vi "Write Optimum Mixer Level for IMD.vi"(10 "Optimum Mixer Level for IMD":T1(array[cluster]), 11 "Spectrum Analyzer in":refnum<class "Spectrum Analyzer.lvclass">) -> (3 "Spectrum Analyzer out":refnum<class "Spectrum Analyzer.lvclass">)   [LabVIEW 2020, in "Spectrum Analyzer.lvclass"]
uses:
  Spectrum Analyzer.lvclass
  Spectrum Analyzer.lvclass/Spectrum Analyzer.ctl
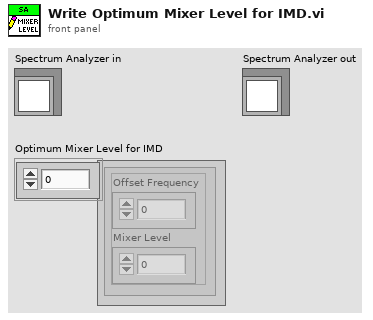
[diagram p1: front panel]
types:
  T1 = cluster{"Offset Frequency":dbl, "Mixer Level":dbl}[]
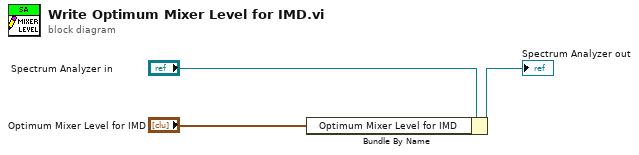
[diagram p0: block diagram]
diagram:
  n1 = Bundle By Name(cluster="Spectrum Analyzer in", "Optimum Mixer Level for IMD"="Optimum Mixer Level for IMD") -> (→"Spectrum Analyzer out":refnum<class "Spectrum Analyzer.lvclass">)
